vi "Update ID.vi"(10 "Debug Data.lvclass":refnum<class "Debug Data.lvclass">, 11 "Debug Log in":refnum<class "Debug Log.lvclass">) -> (2 "Debug Data out":refnum<class "Debug Data.lvclass">, 3 "Debug Log out":refnum<class "Debug Log.lvclass">)   [LabVIEW 2020, in "Debug Log.lvclass"]
uses:
  Debug Log.lvclass
  Debug Data/Debug Data.lvclass
  Debug Log.lvclass/Debug Log.ctl
  Debug Data/Debug Data.lvclass/Debug Data.ctl
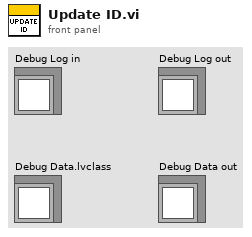
[diagram p1: front panel]
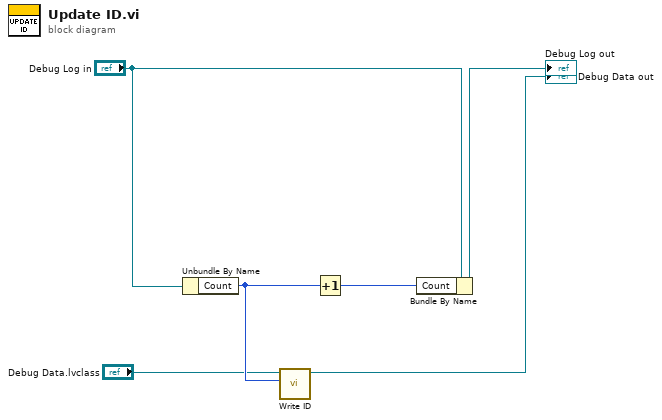
[diagram p0: block diagram]
diagram:
  n1 = Unbundle By Name("Debug Log in") -> ("Count"=w5:u32)
  n2 = call "Write ID.vi"("ID"=w5, "Debug Data in"="Debug Data.lvclass") -> ("Debug Data out"=→"Debug Data out":refnum<class "Debug Data.lvclass">)  [unwired: 8 in, 1 out]
  n3 = Increment(x=w5) -> (x+1=w6:u32)
  n4 = Bundle By Name(cluster="Debug Log in", "Count"=w6) -> (→"Debug Log out":refnum<class "Debug Log.lvclass">)
